vi "Get Topics.vi"(8 "error in":errorcluster, 11 "System in":refnum<class "System.lvclass">) -> (0 "error out":errorcluster, 3 "System out":refnum<class "System.lvclass">)   [LabVIEW 2014, in "System.lvclass"]
uses:
  System.lvclass
  Controls/Topic Ref.ctl
  <vilib>/xml/Close Reference(Node).vi
  <vilib>/xml/Close Reference(NNMap).vi
  <vilib>/xml/NI_XML.lvlib
  <resource>/objmgr/DOMUserDefRef.rc
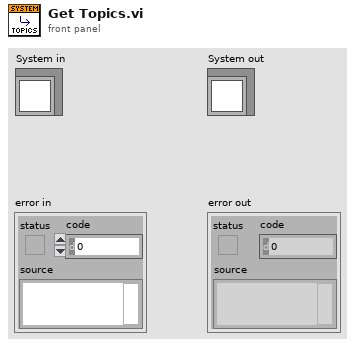
[diagram p1: front panel]
types:
  T1 = typedef "Topic Ref.ctl" = cluster{"Name":string, "Path":path, "Subscribers":string[]}
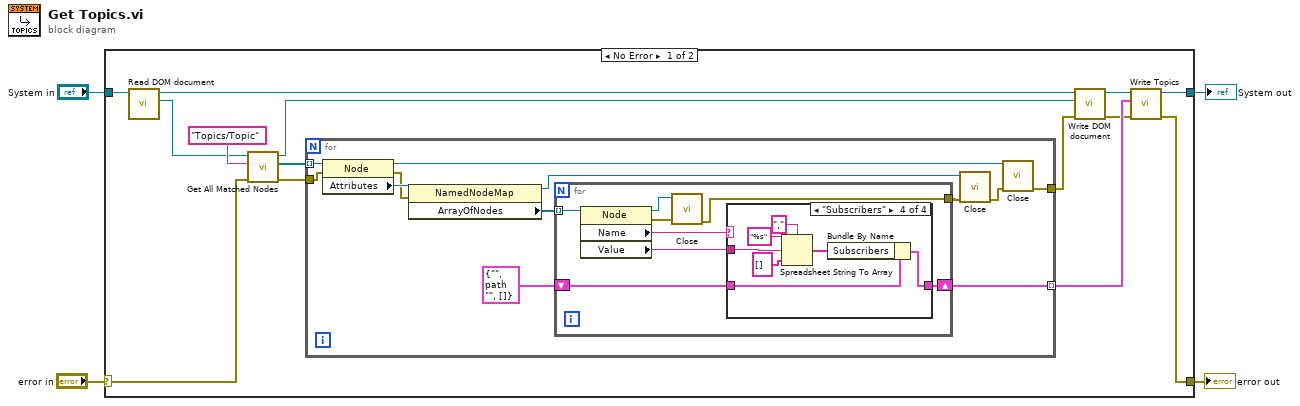
[diagram p0: block diagram]
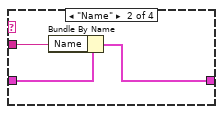
[diagram p3: hidden frame]
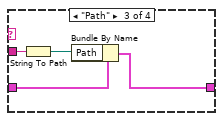
[diagram p4: hidden frame]
diagram:
  n1 = case shown="No Error" "error in" {
    selector: "error in" -> [w17 w55]
    tunnel: [w5 w55] -> w3
    tunnel: [w8 w54] -> w1
    tunnel: "System in" -> [w16 w54]
    frame No Error {
      n2 = call-dynamic "Read DOM document.vi"("System in"=w16) -> ("DOM document"=w11:refnum<k20>, "System out"=w13:refnum<class "System.lvclass">)  [unwired: 8 in, 1 out]
      n3 = call <vilib>:"Get All Matched Nodes.vi"("error in (no error)"=w17, "XPath expression"="Topics/Topic", "node in"=w11) -> ("error out"=w14:errorcluster, "node result array"=w15:refnum<k20>[], "node out"=w10:refnum<k20>)  [unwired: 6 in]
      n4 = for {
        tunnel: w15 -> [w30] mode=indexing
        tunnel: w14 -> [w28]
        tunnel: [w25] -> w7 mode=indexing
        tunnel: [w20] -> w12
        n5 = property class="Node"(reference=w30, error in=w28) -> (reference out=w21:refnum<k20>, error out=w27:errorcluster, "Attributes"=w29:refnum<k20>)
        n6 = property class="NamedNodeMap"(reference=w29, error in=w27) -> (reference out=w23:refnum<k20>, "ArrayOfNodes"=w26:refnum<k20>[])  [unwired: 1 out]
        n7 = for {
          tunnel: w26 -> [w38] mode=indexing
          shift-right: [w32] -> w25
          shift-left: T1 {"Name"="", "Path"=path "", "Subscribers"=[]} ("Topic") -> [w33]
          tunnel: [w31] -> w24
          n8 = property class="Node"(reference=w38) -> (reference out=w36:refnum<k20>, error out=w37:errorcluster, "Name"=w35:string, "Value"=w34:string)  [unwired: 1 in]
          n9 = call-poly <vilib>:"Close.vi"("error in (no error)"=w37, "node"=w36) -> ("error out"=w31:errorcluster)  [unwired: 7 in]
          n10 = case shown="\"Subscribers\"" w35 {
            tunnel: w34 -> [_ w41 w46 w47]
            tunnel: w33 -> [w39 w42 w45 w49]
            tunnel: [w39 w40 w43 w48] -> w32
            frame Default {
              # "Error in config"
            }
            frame "Name" {
              n11 = Bundle By Name(cluster=w42, "Name"=w41) -> (w40:T1)
            }
            frame "Path" {
              n12 = String To Path(string=w46) -> (path=w44:path)
              n13 = Bundle By Name(cluster=w45, "Path"=w44) -> (w43:T1)
            }
            frame "Subscribers" {
              n14 = Spreadsheet String To Array(delimiter (Tab)=",", format string="%s", spreadsheet string=w47, array type (2D Dbl)=string[] []) -> (array=w50:string[])
              n15 = Bundle By Name(cluster=w49, "Subscribers"=w50) -> (w48:T1)
            }
          }
        }
        n16 = call-poly <vilib>:"Close.vi"("error in (no error)"=w24, "named node map"=w23) -> ("error out"=w22:errorcluster)  [unwired: 7 in]
        n17 = call-poly <vilib>:"Close.vi"("error in (no error)"=w22, "node"=w21) -> ("error out"=w20:errorcluster)  [unwired: 7 in]
      }
      n18 = call-dynamic "Write DOM document.vi"("error in"=w12, "DOM document"=w10, "System in"=w13) -> ("error out"=w6:errorcluster, "System out"=w9:refnum<class "System.lvclass">)  [unwired: 7 in]
      n19 = call-dynamic "Write Topics.vi"("error in"=w6, "Topics"=w7, "System in"=w9) -> ("error out"=w5:errorcluster, "System out"=w8:refnum<class "System.lvclass">)  [unwired: 7 in]
    }
    frame Error {
    }
  }
  "error out" <- w3
  "System out" <- w1
